vi "waaca_correcter.vi"(11 "Input weight":dbl) -> (3 "Corrected output weight":dbl)   [LabVIEW 2016]
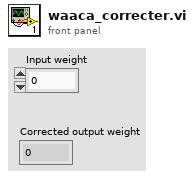
[diagram p1: front panel]
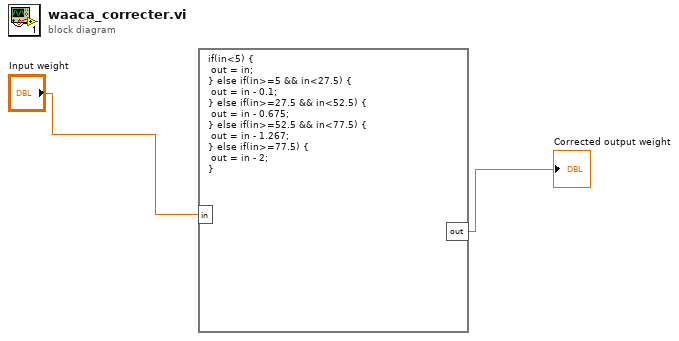
[diagram p0: block diagram]
diagram:
  n1 = formula code="if(in<5) {\n\tout = in;\n} else if(in>=5 && in<27.5) {\n\tout = in - 0.1;\n} else if(in>=27.5 && in<52.5) {\n\tout = in - 0.675;\n} else if(in>=52.5 && in<77.5) {\n\tout = in - 1.267;\n} else if(in>=77.5) {\n\tout = in - 2;\n}"("in"="Input weight") -> ("out"=→"Corrected output weight":dbl)
